vi "Consolidate Errors.vi"(10 "error existing":errorcluster, 11 "error new":errorcluster) -> (0 "error out":errorcluster)   [LabVIEW 2018, in "LTB-1.lvlib" / "3150.lvlib"]
doc: "Merges error from different sources."
uses:
  3150.lvlib
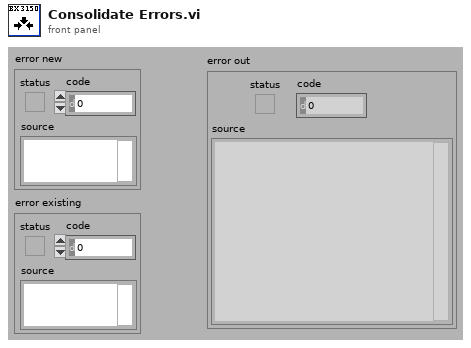
[diagram p1: front panel]
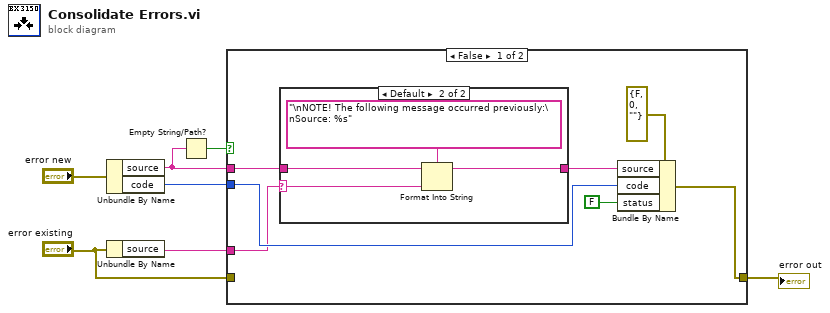
[diagram p0: block diagram]
diagram:
  n1 = Unbundle By Name("error new") -> ("source"=w5:string, "code"=w4:i32)
  n2 = Unbundle By Name("error existing") -> ("source"=w6:string)
  n3 = Empty String/Path?(string/path=w5) -> (empty?=w7:bool)
  n4 = case shown="False" w7 {
    tunnel: "error existing" -> [_ w20]
    tunnel: [w9 w20] -> w1
    tunnel: w4 -> [w14 _]
    tunnel: w6 -> [w12 _]
    tunnel: w5 -> [w11 _]
    frame False {
      n5 = case shown="Default" w12 {
        selector: w12 -> [_ w16]
        tunnel: [w15 w18] -> w13
        tunnel: w11 -> [w15 w17]
        frame "" {
        }
        frame Default {
          n6 = Format Into String(format string="\nNOTE! The following message occurred previously:\nSource: %s", initial string=w17, w16) -> (resulting string=w18:string)  [unwired: 1 in, 1 out]
        }
      }
      n7 = Bundle By Name(cluster=errorcluster {"status"=FALSE, "code"=0, "source"=""} ("error existing"), "source"=w13, "code"=w14, "status"=FALSE) -> (w9:errorcluster)
    }
    frame True {
    }
  }
  "error out" <- w1
